vi "Set Configuration.vi"(8 "error in (no error)":errorcluster, 11 "EST Analog Replay in":refnum<class "EST Analog Replay.lvclass">) -> (0 "error out":errorcluster, 3 "EST Analog Replay out":refnum<class "EST Analog Replay.lvclass">)   [LabVIEW 2015, in "EST Analog Replay.lvclass"]
uses:
  EST Analog Replay.lvclass
  IO Class/Type.ctl
  EST Output/EST Output.lvclass
  IO Class/IO Class.lvclass
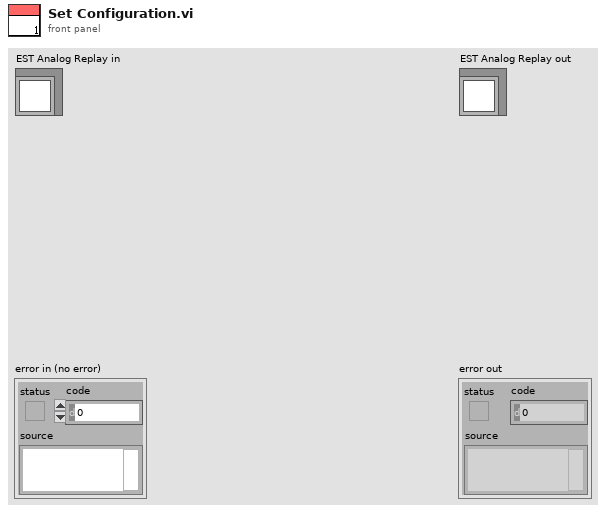
[diagram p1: front panel]
types:
  T1 = typedef "IO Class.lvclass/Type.ctl" = cluster{"Type":string}
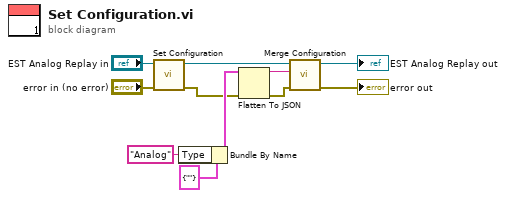
[diagram p0: block diagram]
diagram:
  n1 = call-parent "Set Configuration.vi"("error in (no error)"="error in (no error)", "EST Output in"="EST Analog Replay in") -> ("error out"=w1:errorcluster, "EST Output out"=w3:refnum<class "EST Analog Replay.lvclass">)  [unwired: 8 in]
  n2 = Bundle By Name(cluster=T1 {"Type"=""} ("Type"), "Type"="Analog") -> (w8:T1)
  n3 = Flatten To JSON(anything=w8, error in (no error)=w1) -> (JSON string=w6:string, 11:w5:errorcluster)  [unwired: 1 in]
  n4 = call "Merge Configuration.vi"("error in (no error)"=w5, "Additional Configuration"=w6, "IO Class in"=w3) -> ("error out"=→"error out":errorcluster, "IO Class out"=→"EST Analog Replay out":refnum<class "EST Analog Replay.lvclass">)  [unwired: 7 in]
